vi "Auto Config RC And CRC.vi"(5 "Protected Signal GUID":string="D95BE1B9-793B-430A-998F-7F352C03EC7C", 7 "Counter Value GUID":string="94e87467-031b-484c-a85e-bcbac581524d", 8 "error in (no error)":errorcluster, 10 "Auto Config Setting":T1, 11 "Array":cluster{"Name":string, "Item Ref out":T2}[](array[cluster]) {"Item Ref out" format="%.0x"}) -> (0 "error out":errorcluster)   [LabVIEW 2023, in "Protection and Counter Support System Explorer.lvlib"]
uses:
  Protection and Counter Support System Explorer.lvlib
  <vilib>/NI VeriStand/Custom Device API/Custom Device Item Ref.ctl
  Types/Auto Config Setting.ctl
  <vilib>/NI VeriStand/Custom Device API/Custom Device API.lvlib
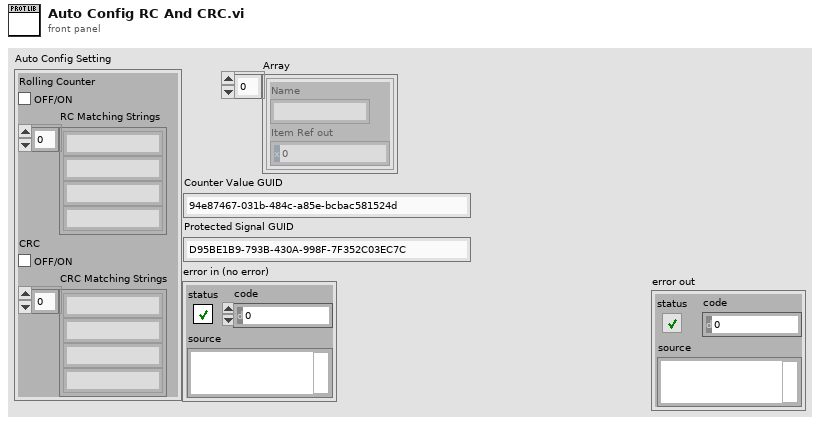
[diagram p1: front panel]
types:
  T1 = typedef "Protection and Counter Support System Explorer.lvlib/Auto Config Setting.ctl" = cluster{"Rolling Counter":bool, "RC Matching Strings":string[], "CRC":bool, "CRC Matching Strings":string[]}
  T2 = typedef "Custom Device API.lvlib/Custom Device Item Ref.ctl" = u64
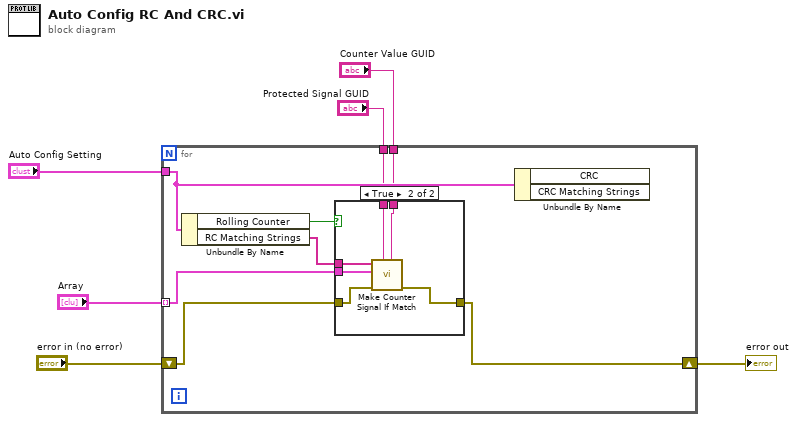
[diagram p0: block diagram]
diagram:
  n1 = for {
    tunnel: "Array" -> [w12] mode=indexing
    tunnel: "Auto Config Setting" -> [w14]
    shift-right: [w9] -> w3
    shift-left: "error in (no error)" -> [w10]
    tunnel: "Protected Signal GUID" -> [w8]
    tunnel: "Counter Value GUID" -> [w7]
    n2 = Unbundle By Name(w14) -> ("Rolling Counter"=w11:bool, "RC Matching Strings"=w13:string[])
    n3 = case shown="True" w11 {
      tunnel: w13 -> [_ w21]
      tunnel: w12 -> [_ w20]
      tunnel: w10 -> [w15 w19]
      tunnel: [w15 w18] -> w9
      tunnel: w8 -> [_ w17]
      tunnel: w7 -> [_ w16]
      frame False {
      }
      frame True {
        n4 = call "Make Counter Signal If Match.vi"("Counter Value GUID"=w16, "Protected Signal GUID"=w17, "error in (no error)"=w19, "Cluster"=w20, "Matching Strings"=w21) -> ("error out"=w18:errorcluster)  [unwired: 6 in]
      }
    }
    n5 = Unbundle By Name(w14) -> ()  [unwired: 2 out]
  }
  "error out" <- w3
